vi "Obtain Broadcast Events.vi"(8 "error in (no error)":errorcluster, 10 "Create New? (F)":bool) -> (0 "error out":errorcluster, 2 "Acquisition Broadcast Events":T1)   [LabVIEW 2019, in "Acquisition.lvlib"]
doc: "This VI Obtains/Creates the Broadcast events that will be used for other modules to register to receive messages from the module that owns this VI.\n\n<b>NOTE</b>: The contents of this VI are automatically generated and modified by the <b>Tools > Delacor > DQMH</b> utilities. Consider using those utilities instead of making your own modifications to this VI.\n_____\nBased on Delacor QMH Project Template 4.0.0.47.\n_____\nBased on DQMH Project Template 6.1.0.94."
uses:
  Acquisition.lvlib
  Broadcast Events--cluster.ctl
  Did Init Argument--cluster.ctl
  Status Updated Argument--cluster.ctl
  Error Reported Argument--cluster.ctl
  Stop Argument--cluster.ctl
  Get Module Execution Status Argument--cluster.ctl
  Acquisition Started Argument--cluster.ctl
  Acquisition Stopped Argument--cluster.ctl
  Data Updated Argument--cluster.ctl
  WiBCI16T_Data.ctl
  WiBCI16T_Status.ctl
  Reg_Map.ctl
  Device Calibrated Argument--cluster.ctl
  Impedance Data Updated Argument--cluster.ctl
  CNV Data Updated Argument--cluster.ctl
  EOC Data Updated Argument--cluster.ctl
panel:
  # "NOTE: The contents of this VI are automatically generated and modified by the Tools > Delacor > DQMH utilities. Consider using those utilities instead of making your own modifications to this VI."
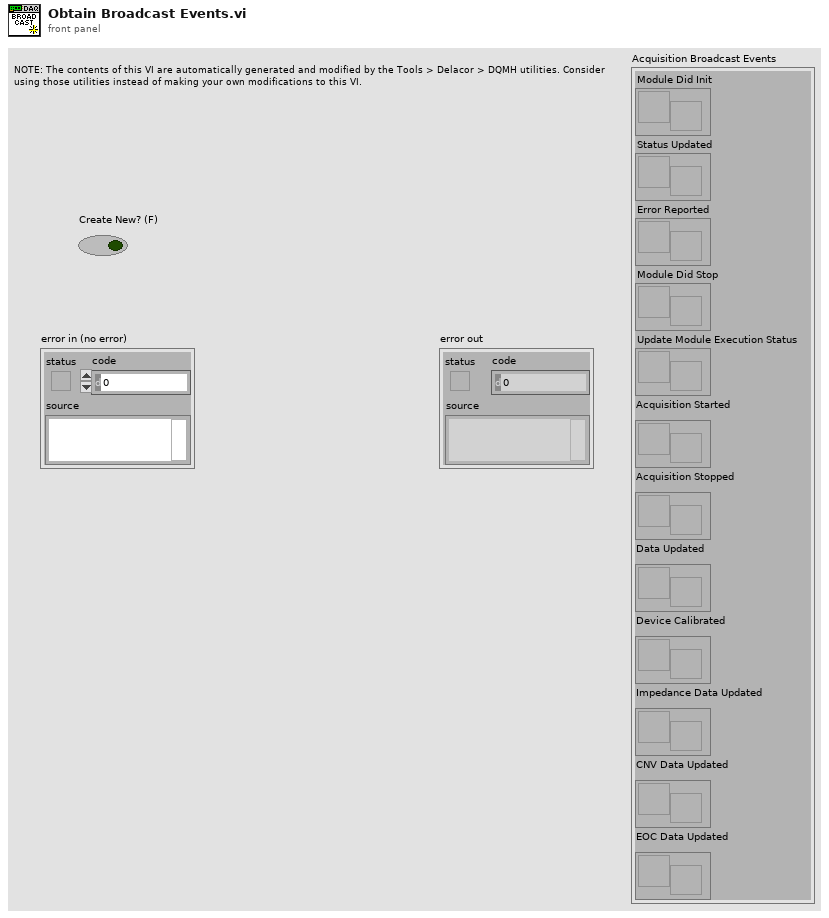
[diagram p1: front panel]
types:
  T1 = typedef "Acquisition.lvlib/Broadcast Events--cluster.ctl" = cluster{"Module Did Init":refnum<user-event>, "Status Updated":refnum<user-event>, "Error Reported":refnum<user-event>, "Module Did Stop":refnum<user-event>, "Update Module Execution Status":refnum<user-event>, "Acquisition Started":refnum<user-event>, "Acquisition Stopped":refnum<user-event>, "Data Updated":refnum<user-event>, "Device Calibrated":refnum<user-event>, "Impedance Data Updated":refnum<user-event>, "CNV Data Updated":refnum<user-event>, "EOC Data Updated":refnum<user-event>}
  T2 = typedef "Acquisition.lvlib/EOC Data Updated Argument--cluster.ctl" = cluster{"WiBCI16T Data":T3, "En MAP":u16}
  T3 = typedef "Acquisition.lvlib/WiBCI16T_Data.ctl" = cluster{"EEG Ch 1":dbl, "EEG Ch 2":dbl, "EEG Ch 3":dbl, "EEG Ch 4":dbl, "EEG Ch 5":dbl, "EEG Ch 6":dbl, "EEG Ch 7":dbl, "EEG Ch 8":dbl, "EEG Ch 9":dbl, "EEG Ch 10":dbl, "EEG Ch 11":dbl, "EEG Ch 12":dbl, "EEG Ch 13":dbl, "EEG Ch 14":dbl, "EEG Ch 15":dbl, "EEG Ch 16":dbl, "X-Accel":i16, "Y-Accel":i16, "Z-Accel":i16, "X-Gyro":i16, "Y-Gyro":i16, "Z-Gyro":i16, "Timer":u32, "Packet ID":u32, "HW Trig1":u8, "SW Trig1":i8, "HW Trig2":u8, "SW Trig2":i8, "WiBCI Status":T4, "Reg Map":T5}
  T4 = typedef "Acquisition.lvlib/WiBCI16T_Status.ctl" = cluster{"Mode Byte":u8, "Ch Config":u8, "Ch Ref Map":u16, "Ch Enable Map":u16, "Temperature":sgl, "Battery":u8, "Version":string}
  T5 = typedef "Acquisition.lvlib/Reg_Map.ctl" = cluster{"ADS1":u8[], "ADS2":u8[]}
  T6 = typedef "Acquisition.lvlib/CNV Data Updated Argument--cluster.ctl" = cluster{"WiBCI16T Data":T3, "En MAP":u16}
  T7 = typedef "Acquisition.lvlib/Impedance Data Updated Argument--cluster.ctl" = cluster{"WiBCI16T Data":T3, "En MAP":u16}
  T8 = typedef "Acquisition.lvlib/Device Calibrated Argument--cluster.ctl" = cluster{"Boolean":bool}
  T9 = typedef "Acquisition.lvlib/Data Updated Argument--cluster.ctl" = cluster{"WiBCI16T Data out":T3, "En MAP":u16}
  T10 = typedef "Acquisition.lvlib/Acquisition Stopped Argument--cluster.ctl" = cluster{"Boolean":bool}
  T11 = typedef "Acquisition.lvlib/Acquisition Started Argument--cluster.ctl" = cluster{"HW ID":string}
  T12 = typedef "Acquisition.lvlib/Get Module Execution Status Argument--cluster.ctl" = cluster{"Running?":bool}
  T13 = typedef "Acquisition.lvlib/Stop Argument--cluster.ctl" = cluster{"Origin":string, "Exit via Stop Module Req?":bool, "Wait for Module to stop?":bool}
  T14 = typedef "Acquisition.lvlib/Error Reported Argument--cluster.ctl" = cluster{"Error":errorcluster, "Additional Information":string, "Module Name":string}
  T15 = typedef "Acquisition.lvlib/Status Updated Argument--cluster.ctl" = cluster{"Status":string}
  T16 = typedef "Acquisition.lvlib/Did Init Argument--cluster.ctl" = cluster{"Init?":bool, "Info":string}
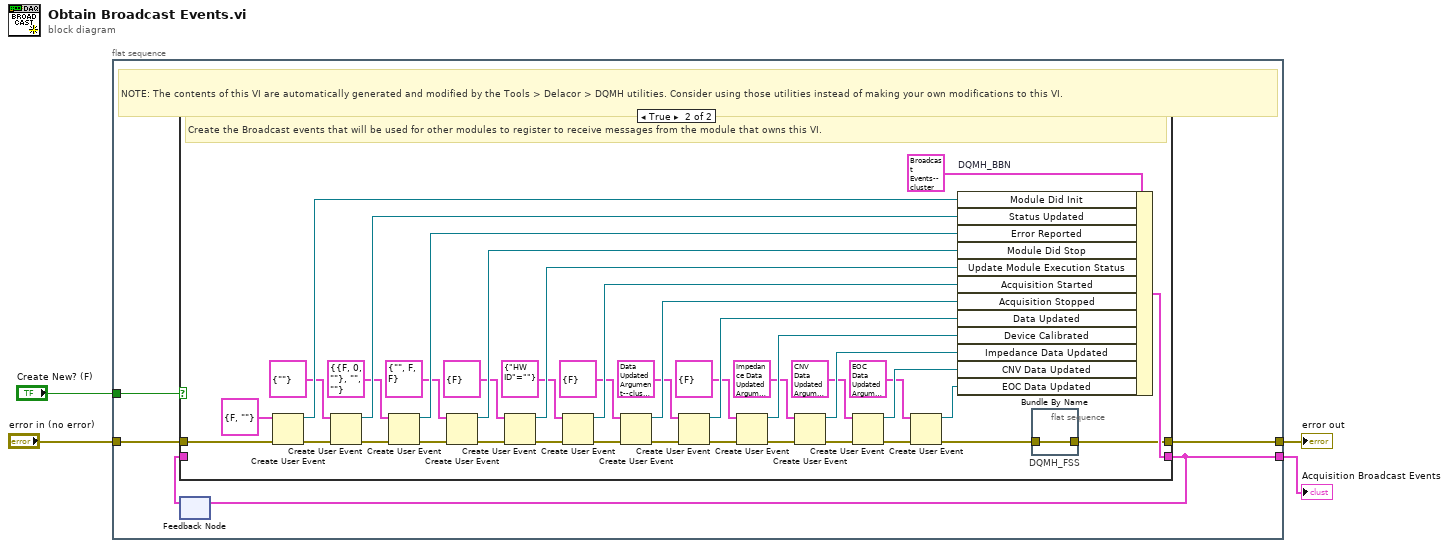
[diagram p0: block diagram]
diagram:
  n1 = flat-sequence {
    tunnel: [w9] -> w4
    tunnel: "error in (no error)" -> [w8]
    tunnel: [w6] -> w2
    tunnel: "Create New? (F)" -> [w5]
    frame #0 {
      # "NOTE: The contents of this VI are automatically generated and modified by the Tools > Delacor > DQMH utilities. Consider using those utilities instead of making your own modifications to this VI."
      n2 = feedback #1() -> (w7:T1)  [unwired: 1 in]
      n3 = case shown="True" w5 {
        tunnel: [w10 w36] -> w9
        tunnel: w8 -> [w10 w51]
        tunnel: [w11 w48] -> w6
        tunnel: w7 -> [w11 _]
        frame False {
          # "Obtain the Broadcast events that were created in a previous call to this VI."
        }
        frame True {
          # "Create the Broadcast events that will be used for other modules to register to receive messages from the module that owns this VI."
          n4 = Create User Event(user event datatype=T16 {"Init?"=FALSE, "Info"=""} ("Did Init Argument"), error in=w51) -> (user event=w49:refnum<user-event>, error out=w46:errorcluster)
          n5 = Create User Event(user event datatype=T15 {"Status"=""} ("Status Updated Argument"), error in=w46) -> (user event=w43:refnum<user-event>, error out=w45:errorcluster)
          n6 = Create User Event(user event datatype=T14 {"Error"={"status"=FALSE, "code"=0, "source"=""}, "Additional Information"="", "Module Name"=""} ("Error Reported Argument"), error in=w45) -> (user event=w40:refnum<user-event>, error out=w42:errorcluster)
          n7 = Create User Event(user event datatype=T13 {"Origin"="", "Exit via Stop Module Req?"=FALSE, "Wait for Module to stop?"=FALSE} ("Stop Argument"), error in=w42) -> (user event=w38:refnum<user-event>, error out=w37:errorcluster)
          n8 = Create User Event(user event datatype=T12 {"Running?"=FALSE} ("Get Module Execution Status Argument"), error in=w37) -> (user event=w34:refnum<user-event>, error out=w35:errorcluster)
          n9 = Create User Event(user event datatype=T11 {"HW ID"=""} ("Acquisition Started Argument"), error in=w35) -> (user event=w31:refnum<user-event>, error out=w32:errorcluster)
          n10 = Create User Event(user event datatype=T10 {"Boolean"=FALSE} ("Acquisition Stopped Argument"), error in=w32) -> (user event=w28:refnum<user-event>, error out=w29:errorcluster)
          n11 = Create User Event(user event datatype=T9 {"WiBCI16T Data out"={"EEG Ch 1"=0.0, "EEG Ch 2"=0.0, "EEG Ch 3"=0.0, "EEG Ch 4"=0.0, "EEG Ch 5"=0.0, "EEG Ch 6"=0.0, "EEG Ch 7"=0.0, "EEG Ch 8"=0.0, "EEG Ch 9"=0.0, "EEG Ch 10"=0.0, "EEG Ch 11"=0.0, "EEG Ch 12"=0.0, "EEG Ch 13"=0.0, "EEG Ch 14"=0.0, "EEG Ch 15"=0.0, "EEG Ch 16"=0.0, "X-Accel"=0, "Y-Accel"=0, "Z-Accel"=0, "X-Gyro"=0, "Y-Gyro"=0, "Z-Gyro"=0, "Timer"=0, "Packet ID"=0, "HW Trig1"=0, "SW Trig1"=0, "HW Trig2"=0, "SW Trig2"=0, "WiBCI Status"={"Mode Byte"=0, "Ch Config"=0, "Ch Ref Map"=0, "Ch Enable Map"=0, "Temperature"=0.0, "Battery"=0, "Version"=""}, "Reg Map"={"ADS1"=[], "ADS2"=[]}}, "En MAP"=0} ("Data Updated Argument"), error in=w29) -> (user event=w25:refnum<user-event>, error out=w26:errorcluster)
          n12 = Create User Event(user event datatype=T8 {"Boolean"=FALSE} ("Device Calibrated Argument"), error in=w26) -> (user event=w22:refnum<user-event>, error out=w23:errorcluster)
          n13 = Create User Event(user event datatype=T7 {"WiBCI16T Data"={"EEG Ch 1"=0.0, "EEG Ch 2"=0.0, "EEG Ch 3"=0.0, "EEG Ch 4"=0.0, "EEG Ch 5"=0.0, "EEG Ch 6"=0.0, "EEG Ch 7"=0.0, "EEG Ch 8"=0.0, "EEG Ch 9"=0.0, "EEG Ch 10"=0.0, "EEG Ch 11"=0.0, "EEG Ch 12"=0.0, "EEG Ch 13"=0.0, "EEG Ch 14"=0.0, "EEG Ch 15"=0.0, "EEG Ch 16"=0.0, "X-Accel"=0, "Y-Accel"=0, "Z-Accel"=0, "X-Gyro"=0, "Y-Gyro"=0, "Z-Gyro"=0, "Timer"=0, "Packet ID"=0, "HW Trig1"=0, "SW Trig1"=0, "HW Trig2"=0, "SW Trig2"=0, "WiBCI Status"={"Mode Byte"=0, "Ch Config"=0, "Ch Ref Map"=0, "Ch Enable Map"=0, "Temperature"=0.0, "Battery"=0, "Version"=""}, "Reg Map"={"ADS1"=[], "ADS2"=[]}}, "En MAP"=0} ("Impedance Data Updated Argument"), error in=w23) -> (user event=w19:refnum<user-event>, error out=w20:errorcluster)
          n14 = Create User Event(user event datatype=T6 {"WiBCI16T Data"={"EEG Ch 1"=0.0, "EEG Ch 2"=0.0, "EEG Ch 3"=0.0, "EEG Ch 4"=0.0, "EEG Ch 5"=0.0, "EEG Ch 6"=0.0, "EEG Ch 7"=0.0, "EEG Ch 8"=0.0, "EEG Ch 9"=0.0, "EEG Ch 10"=0.0, "EEG Ch 11"=0.0, "EEG Ch 12"=0.0, "EEG Ch 13"=0.0, "EEG Ch 14"=0.0, "EEG Ch 15"=0.0, "EEG Ch 16"=0.0, "X-Accel"=0, "Y-Accel"=0, "Z-Accel"=0, "X-Gyro"=0, "Y-Gyro"=0, "Z-Gyro"=0, "Timer"=0, "Packet ID"=0, "HW Trig1"=0, "SW Trig1"=0, "HW Trig2"=0, "SW Trig2"=0, "WiBCI Status"={"Mode Byte"=0, "Ch Config"=0, "Ch Ref Map"=0, "Ch Enable Map"=0, "Temperature"=0.0, "Battery"=0, "Version"=""}, "Reg Map"={"ADS1"=[], "ADS2"=[]}}, "En MAP"=0} ("CNV Data Updated Argument"), error in=w20) -> (user event=w16:refnum<user-event>, error out=w17:errorcluster)
          n15 = Create User Event(user event datatype=T2 {"WiBCI16T Data"={"EEG Ch 1"=0.0, "EEG Ch 2"=0.0, "EEG Ch 3"=0.0, "EEG Ch 4"=0.0, "EEG Ch 5"=0.0, "EEG Ch 6"=0.0, "EEG Ch 7"=0.0, "EEG Ch 8"=0.0, "EEG Ch 9"=0.0, "EEG Ch 10"=0.0, "EEG Ch 11"=0.0, "EEG Ch 12"=0.0, "EEG Ch 13"=0.0, "EEG Ch 14"=0.0, "EEG Ch 15"=0.0, "EEG Ch 16"=0.0, "X-Accel"=0, "Y-Accel"=0, "Z-Accel"=0, "X-Gyro"=0, "Y-Gyro"=0, "Z-Gyro"=0, "Timer"=0, "Packet ID"=0, "HW Trig1"=0, "SW Trig1"=0, "HW Trig2"=0, "SW Trig2"=0, "WiBCI Status"={"Mode Byte"=0, "Ch Config"=0, "Ch Ref Map"=0, "Ch Enable Map"=0, "Temperature"=0.0, "Battery"=0, "Version"=""}, "Reg Map"={"ADS1"=[], "ADS2"=[]}}, "En MAP"=0} ("EOC Data Updated Argument"), error in=w17) -> (user event=w13:refnum<user-event>, error out=w14:errorcluster)
          n16 = Bundle By Name "DQMH_BBN"(cluster=T1 {"Module Did Init"=refnum, "Status Updated"=refnum, "Error Reported"=refnum, "Module Did Stop"=refnum, "Update Module Execution Status"=refnum, "Acquisition Started"=refnum, "Acquisition Stopped"=refnum, "Data Updated"=refnum, "Device Calibrated"=refnum, "Impedance Data Updated"=refnum, "CNV Data Updated"=refnum, "EOC Data Updated"=refnum} ("output cluster"), "Module Did Init"=w49, "Status Updated"=w43, "Error Reported"=w40, "Module Did Stop"=w38, "Update Module Execution Status"=w34, "Acquisition Started"=w31, "Acquisition Stopped"=w28, "Data Updated"=w25, "Device Calibrated"=w22, "Impedance Data Updated"=w19, "CNV Data Updated"=w16, "EOC Data Updated"=w13) -> (w48:T1)
          n17 = flat-sequence "DQMH_FSS" {
            tunnel: w14 -> [w52]
            tunnel: [w52] -> w36
            frame #0 {
            }
          }
        }
      }
      n18 = feedback-in #1(w6) -> ()
    }
  }
  "Acquisition Broadcast Events" <- w2
  "error out" <- w4
